vi "Main_GettingDataC.vi"() -> ()   [LabVIEW 2020]
uses:
  State.ctl
panel:
  out "State":T1=enum."WaitForStart"
  out "error out":errorcluster
  out "Growing":string
  in  "stop":bool
  out "Static Data String":string
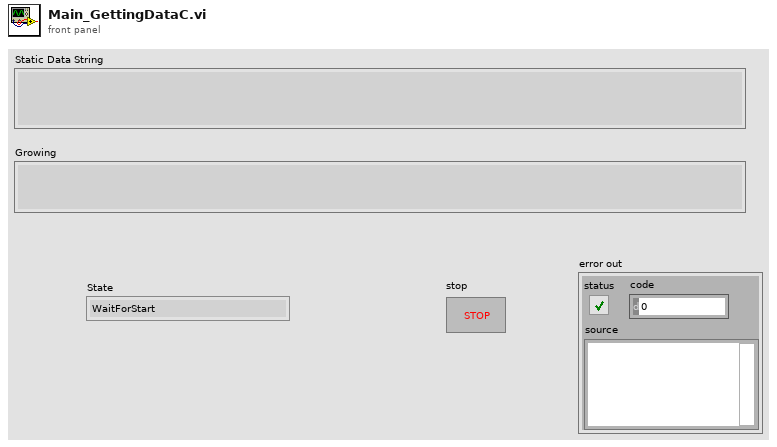
[diagram p1: front panel]
types:
  T1 = typedef "State.ctl" = enum16{"Initialize", "WaitForStart", "Start", "Accumulate", "WaitForEnd", "Cut", "Finalize"}
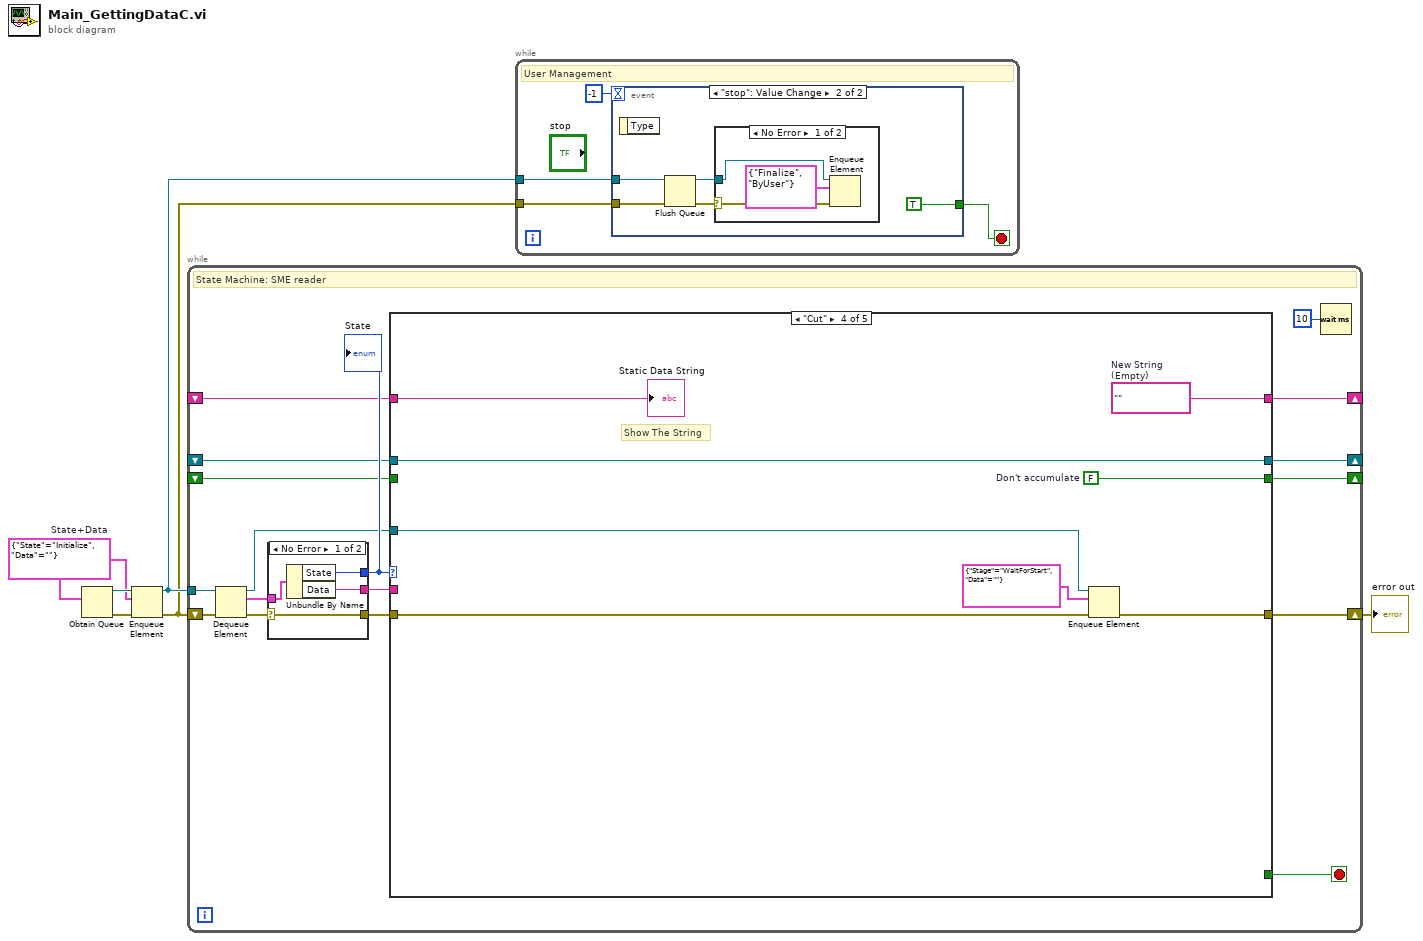
[diagram p0: block diagram]
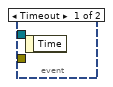
[diagram p2: hidden frame]
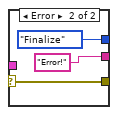
[diagram p4: hidden frame]
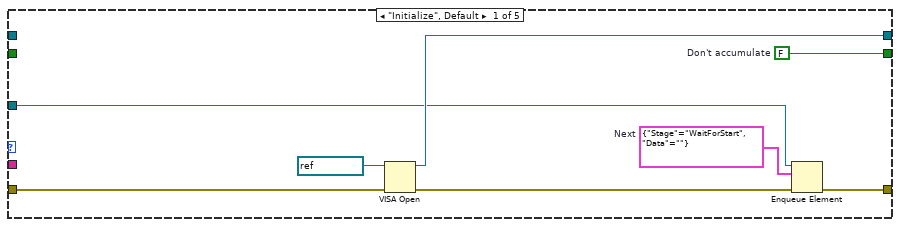
[diagram p5: hidden frame]
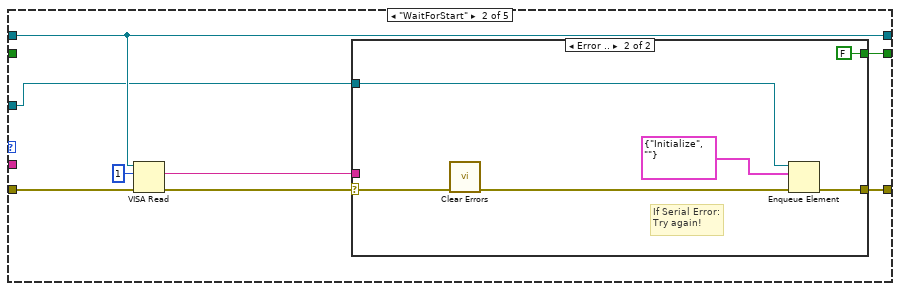
[diagram p6: hidden frame]
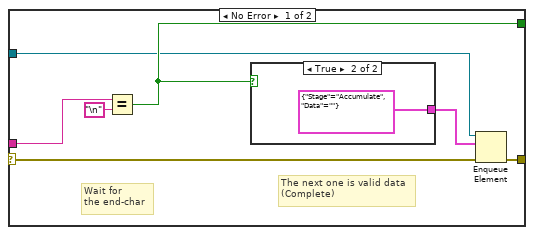
[diagram p7: hidden frame]
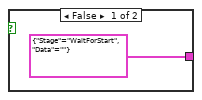
[diagram p8: hidden frame]
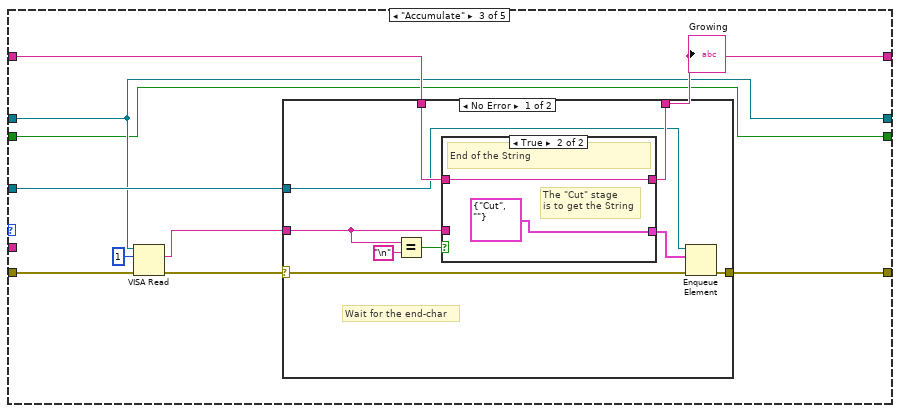
[diagram p9: hidden frame]
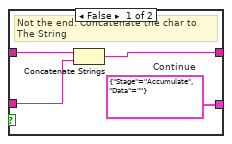
[diagram p10: hidden frame]
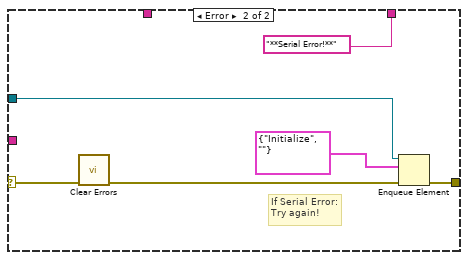
[diagram p11: hidden frame]
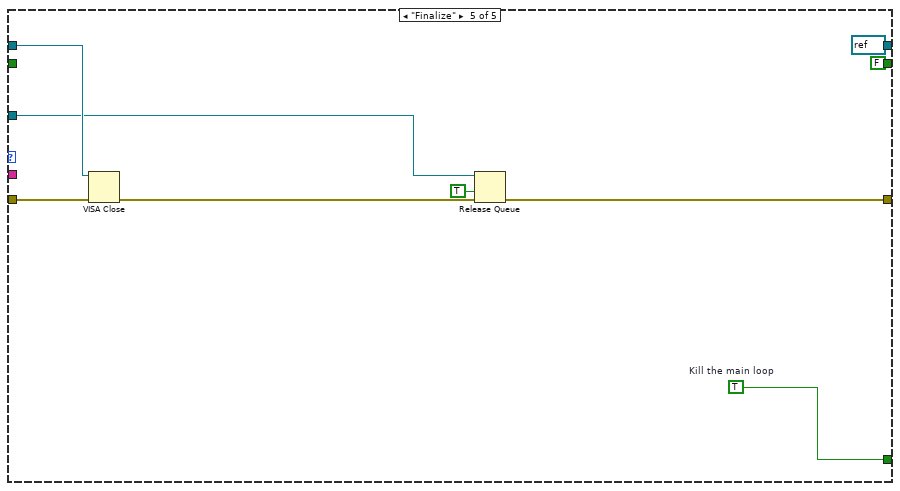
[diagram p12: hidden frame]
diagram:
  w5 = cluster{"State":T1, "Data":string} {"State"=enum."Initialize", "Data"=""}  # State+Data
  n1 = Obtain Queue(element data type=w5) -> (queue out=w6:refnum<queue>, error out=w4:errorcluster)  [unwired: 4 in, 1 out]
  n2 = Enqueue Element(queue=w6, element=w5, error in (no error)=w4) -> (queue out=w3:refnum<queue>, error out=w2:errorcluster)  [unwired: 1 in, 1 out]
  n3 = while {
    shift-right: [w20] -> w1
    shift-left: w2 -> [w12]
    shift-right: [w19] -> _
    shift-left: _ -> [w18]
    shift-right: [w17] -> _
    shift-left: _ -> [w16]
    shift-right: [w14] -> _
    shift-left: _ -> [w15]
    tunnel: w3 -> [w13]
    stop <- w9 stop-if-true
    # "State Machine: SME reader"
    n4 = Dequeue Element(queue=w13, error in (no error)=w12) -> (queue out=w8:refnum<queue>, element=w10:cluster{"State":T1, "Data":string}, error out=w11:errorcluster)  [unwired: 1 in, 1 out]
    n5 = case shown="No Error" w11 {
      selector: w11 -> [w24 w28]
      tunnel: w10 -> [w27 _]
      tunnel: [w26 State."Finalize" ("Stage")] -> w23
      tunnel: [w25 "Error!" ("Data")] -> w22
      tunnel: [w24 w28] -> w21
      frame No Error {
        n6 = Unbundle By Name(w27) -> ("State"=w26:T1, "Data"=w25:string)
      }
      frame Error {
      }
    }
    "State" <- w23
    n7 = case shown="\"Cut\"" w23 {
      tunnel: w22 -> [_ _ _ _ _]
      tunnel: w21 -> [w38 w45 w70 w95 w108]
      tunnel: [w31 w40 w65 w94 w104] -> w20
      tunnel: [w37 w42 w64 w99 refnum<visa-resource-name> refnum ("VISA resource name")] -> w19
      tunnel: w18 -> [_ w42 w64 w99 w109]
      tunnel: [w35 w43 w63 w93 FALSE ("Don't accumulate")] -> w17
      tunnel: w16 -> [_ _ w63 _ _]
      tunnel: w15 -> [_ _ w69 w100 _]
      tunnel: [_ _ w67 w98 _] -> w14
      tunnel: [_ _ _ _ w105] -> w9
      tunnel: w8 -> [w34 w41 w66 w97 w103]
      frame "Initialize", Default {
        w35 = FALSE  # Don't accumulate
        w33 = cluster{"Stage":T1, "Data":string} {"Stage"=enum."WaitForStart", "Data"=""}  # Next
        n8 = VISA Open(error in (no error)=w38, VISA resource name=refnum<visa-resource-name> "CNCB0") -> (VISA resource name=w37:refnum<visa-resource-name>, error out=w32:errorcluster)  [unwired: 3 in]
        n9 = Enqueue Element(queue=w34, element=w33, error in (no error)=w32) -> (error out=w31:errorcluster)  [unwired: 1 in, 2 out]
      }
      frame "WaitForStart" {
        n10 = VISA Read(VISA resource name=w42, byte count=u32 1, error in (no error)=w45) -> (read buffer=w44:string, error out=w39:errorcluster)  [unwired: 2 out]
        n11 = case shown="Error .." w39 {
          selector: w39 -> [w47 w57]
          tunnel: w44 -> [w53 _]
          tunnel: [w51 FALSE] -> w43
          tunnel: w41 -> [w50 w61]
          tunnel: [w49 w59] -> w40
          frame No Error {
            # "The next one is valid data\n(Complete)"
            # "Wait for \nthe end-char"
            n12 = Equal?(x=w53, y="\n") -> (x = y?=w51:bool)
            n13 = case shown="True" w51 {
              tunnel: [cluster{"Stage":T1, "Data":string} {"Stage"=enum."WaitForStart", "Data"=""} ("Next") cluster{"Stage":T1, "Data":string} {"Stage"=enum."Accumulate", "Data"=""} ("Next")] -> w48
              frame False {
              }
              frame True {
              }
            }
            n14 = Enqueue Element(queue=w50, element=w48, error in (no error)=w47) -> (error out=w49:errorcluster)  [unwired: 1 in, 2 out]
          }
          frame Error {
            # "If Serial Error:\nTry again!"
            n15 = call <vilib>:"Clear Errors.vi"("error in (no error)"=w57) -> ("error out"=w56:errorcluster)  [unwired: 5 in, 1 out]
            n16 = Enqueue Element(queue=w61, element=cluster{"Stage":T1, "Data":string} {"Stage"=enum."Initialize", "Data"=""}, error in (no error)=w56) -> (error out=w59:errorcluster)  [unwired: 1 in, 2 out]
          }
        }
      }
      frame "Accumulate" {
        n17 = VISA Read(VISA resource name=w64, byte count=u32 1, error in (no error)=w70) -> (read buffer=w68:string, error out=w62:errorcluster)  [unwired: 2 out]
        n18 = case shown="No Error" w62 {
          selector: w62 -> [w72 w88]
          tunnel: w69 -> [w79 _]
          tunnel: w68 -> [w78 _]
          tunnel: [w77 "**Serial Error!**" ("New String\n(Empty)")] -> w67
          tunnel: w66 -> [w75 w90]
          tunnel: [w74 w91] -> w65
          frame No Error {
            # "Wait for the end-char"
            n19 = Equal?(x=w78, y="\n") -> (x = y?=w73:bool)
            n20 = case shown="True" w73 {
              tunnel: [w84 cluster{"Stage":T1, "Data":string} {"Stage"=enum."Cut", "Data"=""} ("Next")] -> w76
              tunnel: w79 -> [w83 w86]
              tunnel: w78 -> [w82 _]
              tunnel: [w81 w86] -> w77
              frame False {
                w84 = cluster{"Stage":T1, "Data":string} {"Stage"=enum."Accumulate", "Data"=""}  # Continue
                # "Not the end: Concatenate the char to The String"
                n21 = Concatenate Strings(w83, w82) -> (w81:string)
              }
              frame True {
                # "The \"Cut\" stage\nis to get the String"
                # "End of the String"
              }
            }
            n22 = Enqueue Element(queue=w75, element=w76, error in (no error)=w72) -> (error out=w74:errorcluster)  [unwired: 1 in, 2 out]
          }
          frame Error {
            # "If Serial Error:\nTry again!"
            n23 = call <vilib>:"Clear Errors.vi"("error in (no error)"=w88) -> ("error out"=w87:errorcluster)  [unwired: 5 in, 1 out]
            n24 = Enqueue Element(queue=w90, element=cluster{"Stage":T1, "Data":string} {"Stage"=enum."Initialize", "Data"=""}, error in (no error)=w87) -> (error out=w91:errorcluster)  [unwired: 1 in, 2 out]
          }
        }
        "Growing" <- w67
      }
      frame "Cut" {
        w93 = FALSE  # Don't accumulate
        w98 = ""  # New String (Empty)
        # "Show The String"
        n25 = Enqueue Element(queue=w97, element=cluster{"Stage":T1, "Data":string} {"Stage"=enum."WaitForStart", "Data"=""} ("Next"), error in (no error)=w95) -> (error out=w94:errorcluster)  [unwired: 1 in, 2 out]
        "Static Data String" <- w100
      }
      frame "Finalize" {
        w105 = TRUE  # Kill the main loop
        n26 = VISA Close(VISA resource name=w109, error in (no error)=w108) -> (error out=w102:errorcluster)
        n27 = Release Queue(queue=w103, force destroy? (F)=TRUE, error in (no error)=w102) -> (error out=w104:errorcluster)  [unwired: 2 out]
      }
    }
    n28 = Wait (ms)(milliseconds to wait=u32 10) -> ()  [unwired: 1 out]
  }
  "error out" <- w1
  n29 = while {
    tunnel: w3 -> [w111]
    tunnel: w2 -> [w110]
    stop <- w112 stop-if-true
    # "User Management"
    n30 = event shown="[1] \"stop\": Value Change" {
      selector: _ -> [_ _]
      dyn-events: _ -> [_ _]
      timeout: -1 -> [_ _]
      tunnel: [_ TRUE] -> w112
      tunnel: w111 -> [_ w116]
      tunnel: w110 -> [_ w117]
      event Timeout {
        n31 = event-data() -> ()  [unwired: 1 in, 1 out]
      }
      event "stop": Value Change {
        n32 = event-data() -> ()  [unwired: 1 in, 1 out]
        n33 = Flush Queue(queue=w116, error in (no error)=w117) -> (queue out=w115:refnum<queue>, error out=w114:errorcluster)  [unwired: 1 out]
        n34 = case shown="No Error" w114 {
          selector: w114 -> [w119 _]
          tunnel: w115 -> [w120 _]
          frame No Error {
            n35 = Enqueue Element(queue=w120, element=cluster{"Stage":T1, "Data":string} {"Stage"=enum."Finalize", "Data"="ByUser"}, error in (no error)=w119) -> ()  [unwired: 1 in, 3 out]
          }
          frame Error {
            # "Already dead"
          }
        }
      }
    }
  }
